vi "PCO_GetModulationMode.vi"(8 "error in (no error)":errorcluster {"code" format="%x"}, 11 "ph":u64) -> (0 "error out":errorcluster {"code" format="%x"}, 1 "wModulationMode":u16(ring) items=["OFF", "ON"], 2 "ErrorMessage":i32 format="%x", 3 "ph out":u64, 4 "wTimebasePeriodical":u16(ring) items=["ns", "us", "ms"], 5 "dwPeriodicalTime":u32, 6 "lMonitorOffset":i32, 7 "dwNumberOfExposures":u32)   [LabVIEW 2020, in "SDK.lvlib" / "TimingControl.lvlib"]
doc: "<b>Description:</b>\nThis function returns the current settings of the modulation mode and its corresponding parameters.\n\nThe modulation mode is an optional feature which is not available for all camera models. To determine if modulation mode is available first check if second descriptor is loadable through flag ENHANCED_DESCRIPTOR_2 in dwGeneralCapsDESC1 of PCO_Description structure. Then the presence of flag MODULATE in dwModulateCapsDESC2 of PCO_Description2 structure must be checked.\n\n<b>Supported camera type:</b>\nAvailable for special versions of pco.1600, pco.2000 and pco.4000.\n\n<b>Descriptor dependency:</b>\ndwGeneralCapsDESC1: ENHANCED_DESCRIPTOR_2\ndwModulateCapsDESC2: MODULATE"
uses:
  TimingControl.lvlib
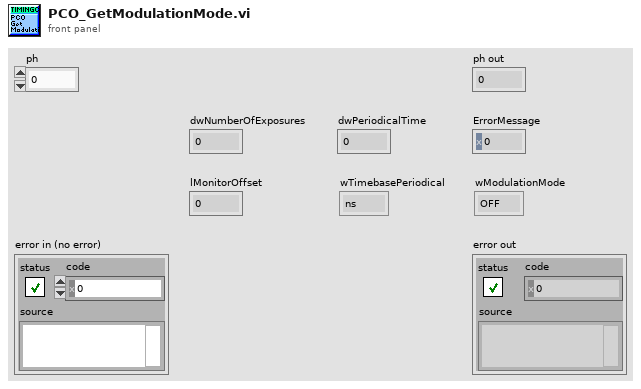
[diagram p1: front panel]
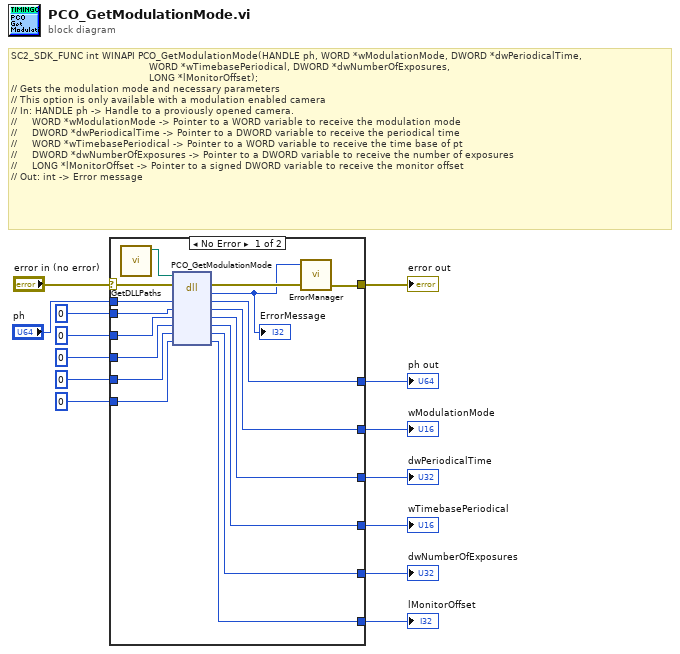
[diagram p0: block diagram]
diagram:
  # "SC2_SDK_FUNC int WINAPI PCO_GetModulationMode(HANDLE ph, WORD *wModulationMode, DWORD *dwPeriodicalTime,\n                                              WORD *wTimebasePeriodical, DWORD *dwNumberOfExposures,\n                                              LONG *lMonitorOffset);\n// Gets the modulation mode and necessary parameters\n// This option is only available with a modulation enabled camera\n// In: HANDLE ph -> Handle to a proviously opened camera.\n//     WORD *wModulationMode -> Pointer to a WORD variable to receive the modulation mode\n//     DWORD *dwPeriodicalTime -> Pointer to a DWORD variable to receive the periodical time\n//     WORD *wTimebasePeriodical -> Pointer to a WORD variable to receive the time base of pt\n//     DWORD *dwNumberOfExposures -> Pointer to a DWORD variable to receive the number of exposures\n//     LONG *lMonitorOffset -> Pointer to a signed DWORD variable to receive the monitor offset\n// Out: int -> Error message"
  n1 = case shown="No Error" "error in (no error)" {
    selector: "error in (no error)" -> [w19 w38]
    tunnel: "ph" -> [w31 w37]
    tunnel: [w30 w37] -> w13
    tunnel: u16 0 ("wModulationMode") -> [w29 w36]
    tunnel: [w28 w36] -> w11
    tunnel: u32 0 ("dwPeriodicalTime") -> [w27 w35]
    tunnel: [w26 w35] -> w9
    tunnel: u16 0 ("wTimebasePeriodical") -> [w25 w34]
    tunnel: [w24 w34] -> w7
    tunnel: u32 0 ("dwNumberOfExposures") -> [w23 w33]
    tunnel: [w22 w33] -> w5
    tunnel: 0 ("lMonitorOffset") -> [w21 w32]
    tunnel: [w20 w32] -> w3
    tunnel: [w17 w38] -> w2
    frame No Error {
      n2 = call "GetDLLPaths.vi"() -> ("SC2_Cam_Path"=w15:path)  [unwired: 9 in, 2 out]
      n3 = dll-call lib="?" fn="PCO_GetModulationMode"(path in=w15, error in=w19, "ph"=w31, "wModulationMode"=w29, "dwPeriodicalTime"=w27, "wTimebasePeriodical"=w25, "dwNumberOfExposures"=w23, "lMonitorOffset"=w21) -> (error out=w18:errorcluster, "return type"=w16:i32, "ph"=w30:u64, "wModulationMode"=w28:u16, "dwPeriodicalTime"=w26:u32, "wTimebasePeriodical"=w24:u16, "dwNumberOfExposures"=w22:u32, "lMonitorOffset"=w20:i32)  [unwired: 1 in, 1 out]
      "ErrorMessage" <- w16
      n4 = call "ErrorManager.vi"("error in (no error)"=w18, "error code"=w16) -> ("error out"=w17:errorcluster)  [unwired: 3 in]
    }
    frame Error {
    }
  }
  "ph out" <- w13
  "wModulationMode" <- w11
  "dwPeriodicalTime" <- w9
  "wTimebasePeriodical" <- w7
  "dwNumberOfExposures" <- w5
  "lMonitorOffset" <- w3
  "error out" <- w2
